vi "MAIN CARICA STRINGHE.vi"() -> ()   [LabVIEW 2019]
uses:
  <vilib>/Utility/file.llb/Read Delimited Spreadsheet (string).vi
panel:
  out "Array":string[](array[string])
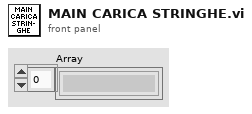
[diagram p1: front panel]
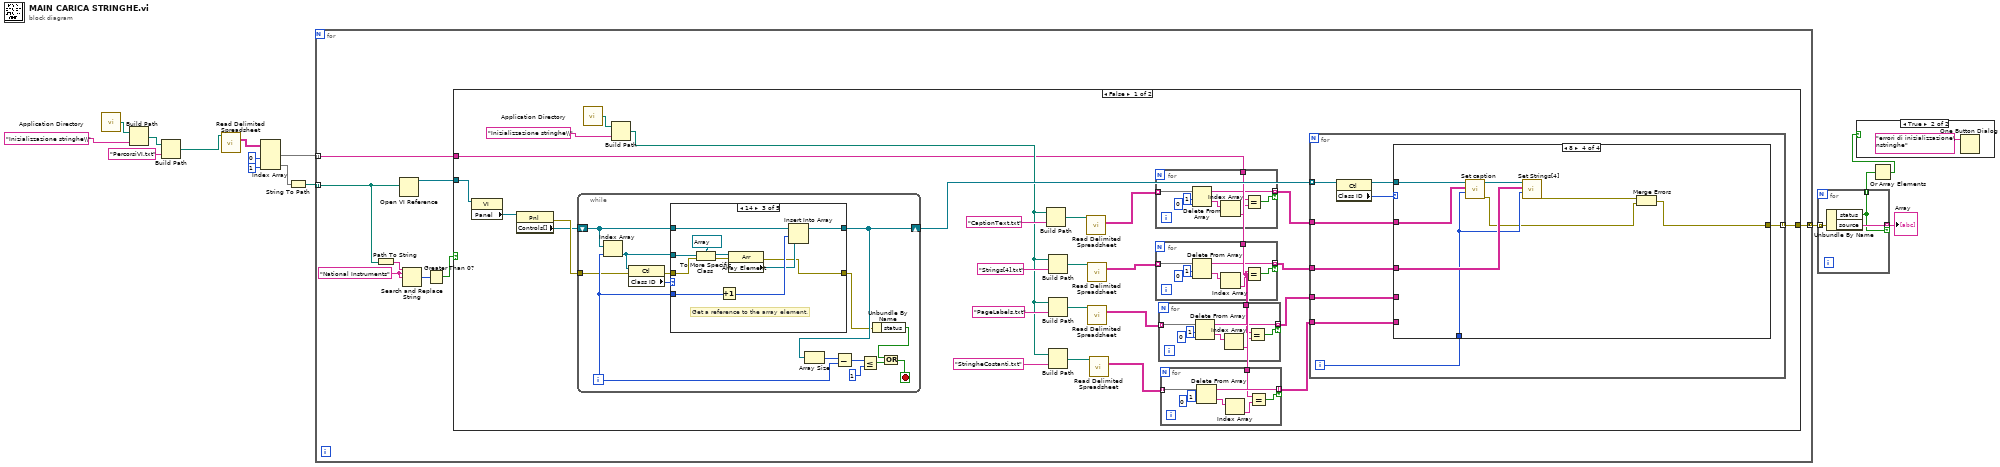
[diagram p0: block diagram]
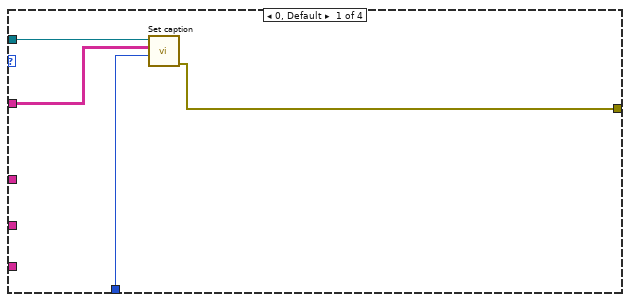
[diagram p3: hidden frame]
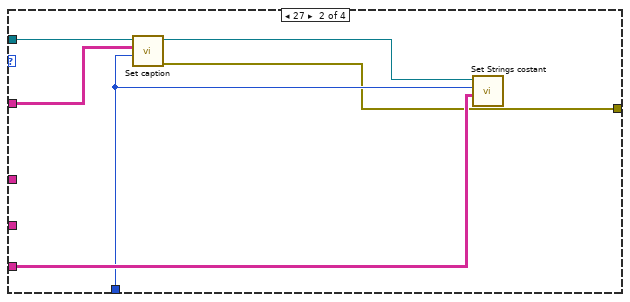
[diagram p4: hidden frame]
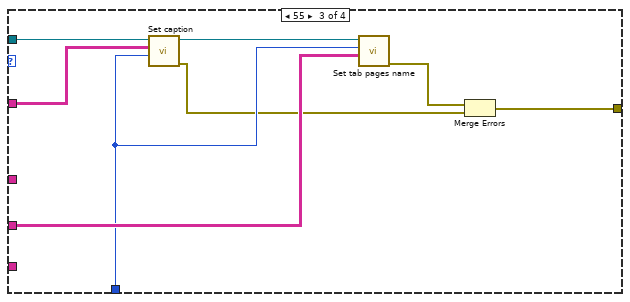
[diagram p5: hidden frame]
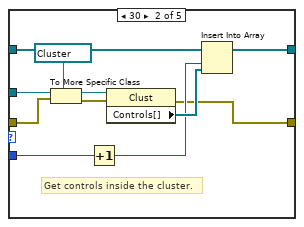
[diagram p7: hidden frame]
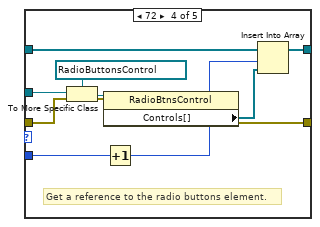
[diagram p8: hidden frame]
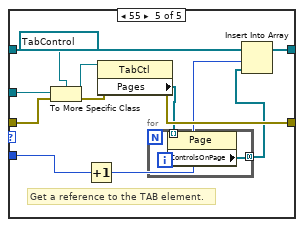
[diagram p9: hidden frame]
diagram:
  n1 = call <vilib>:"Application Directory.vi"() -> ("Application Directory"=w4:path)
  n2 = Build Path(base path=w4, name or relative path="Inizializzazione stringhe\\") -> (appended path=w5:path)
  n3 = Build Path(base path=w5, name or relative path="PercorsiVI.txt") -> (appended path=w6:path)
  n4 = call-poly <vilib>:"Read Delimited Spreadsheet.vi"("file path (dialog if empty)"=w6) -> ("all rows"=w7:string[][])  [unwired: 9 in, 5 out]
  n5 = Index Array(array=w7, index (col) #1=0 ("disabled index (col)"), index (col) #2=1 ("index (col)")) -> (element #1=w10:string[], element #2=w11:string[])  [unwired: 2 in]
  n6 = String To Path(string=w11) -> (path=w12:path[])
  n7 = for {
    tunnel: w12 -> [w21] mode=indexing
    tunnel: w10 -> [w22] mode=indexing
    tunnel: [w16] -> w15 mode=concatenating
    w19 = "National Instruments" ("search string")
    n8 = Path To String(path=w21) -> (string=w20:string)
    n9 = Open VI Reference(vi path=w21) -> (vi reference=w23:refnum<vi>)  [unwired: 5 in, 1 out]
    n10 = Search and Replace String(input string=w20, search string=w19, replace string=w19) -> (number of replacements=w18:i32)  [unwired: 5 in, 3 out]
    n11 = Greater Than 0?(x=w18) -> (x > 0?=w17:bool)
    n12 = case shown="False" w17 {
      tunnel: w23 -> [w46 _]
      tunnel: w22 -> [w24 _]
      tunnel: [w25 _] -> w16
      frame False {
        n13 = property class="VI"(reference=w46) -> ("Panel"=w47:refnum<vi>)  [unwired: 1 in, 2 out]
        n14 = property class="Pnl"(reference=w47) -> (error out=w49:errorcluster, "Controls[]"=w48:refnum<vi>[])  [unwired: 1 in, 1 out]
        n15 = while {
          shift-right: [w121] -> w37
          shift-left: w48 -> [w122]
          tunnel: w49 -> [w120]
          i -> [w127]
          stop <- w125 stop-if-true
          n16 = Index Array(array=w122, index=w127) -> (element=w123:refnum<vi>)
          n17 = property class="Ctl"(reference=w123, error in=w120) -> (error out=w119:errorcluster, "Class ID"=w124:u32)  [unwired: 1 out]
          n18 = case shown="14" w124 {
            tunnel: w123 -> [_ w143 w154 w165 w177]
            tunnel: w122 -> [w132 w140 w151 w164 w176]
            tunnel: w127 -> [_ w139 w150 w163 w175]
            tunnel: [w132 w137 w149 w162 w174] -> w121
            tunnel: w119 -> [w131 w135 w146 w161 w173]
            tunnel: [w131 w133 w144 w160 w172] -> w117
            frame 0, Default {
            }
            frame 30 {
              # "Get controls inside the cluster."
              n19 = To More Specific Class(target class=refnum<vi> refnum ("target class 3"), reference=w143, error in=w135) -> (specific class reference=w142:refnum<vi>, error out=w134:errorcluster)
              n20 = Increment(x=w139) -> (x+1=w136:i32)
              n21 = property class="Clust"(reference=w142, error in=w134) -> (error out=w133:errorcluster, "Controls[]"=w138:refnum<vi>[])  [unwired: 1 out]
              n22 = Insert Into Array(array=w140, index=w136, new element=w138) -> (w137:refnum<vi>[])
            }
            frame 14 {
              # "Get a reference to the array element."
              n23 = To More Specific Class(target class=refnum<vi> refnum ("target class 4"), reference=w154, error in=w146) -> (specific class reference=w153:refnum<vi>, error out=w145:errorcluster)
              n24 = Increment(x=w150) -> (x+1=w148:i32)
              n25 = property class="Arr"(reference=w153, error in=w145) -> (error out=w144:errorcluster, "Array Element"=w147:refnum<vi>)  [unwired: 1 out]
              n26 = Insert Into Array(array=w151, index=w148, new element=w147) -> (w149:refnum<vi>[])
            }
            frame 72 {
              # "Get a reference to the radio buttons element."
              n27 = To More Specific Class(target class=refnum<vi> refnum ("Calcolo P2"), reference=w165, error in=w161) -> (specific class reference=w159:refnum<vi>, error out=w156:errorcluster)
              n28 = property class="RadioBtnsControl"(reference=w159, error in=w156) -> (error out=w160:errorcluster, "Controls[]"=w157:refnum<vi>[])  [unwired: 1 out]
              n29 = Increment(x=w163) -> (x+1=w158:i32)
              n30 = Insert Into Array(array=w164, index=w158, new element=w157) -> (w162:refnum<vi>[])
            }
            frame 55 {
              # "Get a reference to the TAB element."
              n31 = To More Specific Class(target class=refnum<vi> refnum ("Tab Control"), reference=w177, error in=w173) -> (specific class reference=w171:refnum<vi>, error out=w169:errorcluster)
              n32 = Increment(x=w175) -> (x+1=w170:i32)
              n33 = property class="TabCtl"(reference=w171, error in=w169) -> (error out=w172:errorcluster, "Pages"=w167:refnum<vi>[])  [unwired: 1 out]
              n34 = for {
                tunnel: w167 -> [w179] mode=indexing
                tunnel: [w178] -> w166 mode=concatenating
                n35 = property class="Page"(reference=w179) -> ("ControlsOnPage"=w178:refnum<vi>[])  [unwired: 1 in, 2 out]
              }
              n36 = Insert Into Array(array=w176, index=w170, new element=w166) -> (w174:refnum<vi>[])
            }
          }
          n37 = Array Size(array=w121) -> (size(s)=w130:i32)
          n38 = Subtract(x=w130, y=w127) -> (x-y=w129:i32)
          n39 = Less Or Equal?(x=w129, y=1) -> (x <= y?=w126:bool)
          n40 = Unbundle By Name(w117) -> ("status"=w118:bool)
          n41 = Or(x=w118, y=w126) -> (x .or. y?=w125:bool)
        }
        n42 = call <vilib>:"Application Directory.vi"() -> ("Application Directory"=w27:path)
        n43 = Build Path(base path=w27, name or relative path="Inizializzazione stringhe\\") -> (appended path=w26:path)
        n44 = Build Path(base path=w26, name or relative path="CaptionText.txt") -> (appended path=w45:path)
        n45 = Build Path(base path=w26, name or relative path="Strings[4].txt") -> (appended path=w40:path)
        n46 = Build Path(base path=w26, name or relative path="PageLabels.txt") -> (appended path=w39:path)
        n47 = Build Path(base path=w26, name or relative path="StringheCostanti.txt") -> (appended path=w38:path)
        n48 = call-poly <vilib>:"Read Delimited Spreadsheet.vi"("file path (dialog if empty)"=w45) -> ("all rows"=w36:string[][])  [unwired: 9 in, 5 out]
        n49 = call-poly <vilib>:"Read Delimited Spreadsheet.vi"("file path (dialog if empty)"=w40) -> ("all rows"=w34:string[][])  [unwired: 9 in, 5 out]
        n50 = call-poly <vilib>:"Read Delimited Spreadsheet.vi"("file path (dialog if empty)"=w39) -> ("all rows"=w33:string[][])  [unwired: 9 in, 5 out]
        n51 = call-poly <vilib>:"Read Delimited Spreadsheet.vi"("file path (dialog if empty)"=w38) -> ("all rows"=w32:string[][])  [unwired: 9 in, 5 out]
        n52 = for {
          tunnel: w36 -> [w81] mode=indexing
          tunnel: [w77] -> w35 mode=indexing if=w75
          tunnel: w24 -> [w74]
          n53 = Delete From Array(array=w81, length=1, index=0) -> (deleted portion=w78:string[], array with subset deleted=w77:string[])
          n54 = Index Array(array=w78) -> (element=w76:string)  [unwired: 1 in]
          n55 = Equal?(x=w74, y=w76) -> (x = y?=w75:bool)
        }
        n56 = for {
          tunnel: w34 -> [w73] mode=indexing
          tunnel: [w69] -> w31 mode=indexing if=w67
          tunnel: w24 -> [w66]
          n57 = Delete From Array(array=w73, length=1, index=0) -> (deleted portion=w70:string[], array with subset deleted=w69:string[])
          n58 = Index Array(array=w70) -> (element=w68:string)  [unwired: 1 in]
          n59 = Equal?(x=w66, y=w68) -> (x = y?=w67:bool)
        }
        n60 = for {
          tunnel: w33 -> [w65] mode=indexing
          tunnel: [w61] -> w30 mode=indexing if=w59
          tunnel: w24 -> [w58]
          n61 = Delete From Array(array=w65, length=1, index=0) -> (deleted portion=w62:string[], array with subset deleted=w61:string[])
          n62 = Index Array(array=w62) -> (element=w60:string)  [unwired: 1 in]
          n63 = Equal?(x=w58, y=w60) -> (x = y?=w59:bool)
        }
        n64 = for {
          tunnel: w32 -> [w57] mode=indexing
          tunnel: [w53] -> w29 mode=indexing if=w51
          tunnel: w24 -> [w50]
          n65 = Delete From Array(array=w57, length=1, index=0) -> (deleted portion=w54:string[], array with subset deleted=w53:string[])
          n66 = Index Array(array=w54) -> (element=w52:string)  [unwired: 1 in]
          n67 = Equal?(x=w50, y=w52) -> (x = y?=w51:bool)
        }
        n68 = for {
          tunnel: w35 -> [w87]
          tunnel: w31 -> [w86]
          tunnel: w37 -> [w90] mode=indexing
          tunnel: w30 -> [w84]
          tunnel: w29 -> [w83]
          tunnel: [w82] -> w25 mode=indexing
          i -> [w85]
          n69 = property class="Ctl"(reference=w90) -> (reference out=w88:refnum<vi>, "Class ID"=w89:u32)  [unwired: 1 in, 1 out]
          n70 = case shown="8" w89 {
            tunnel: w88 -> [w94 w100 w108 w115]
            tunnel: w87 -> [w93 w99 w107 w113]
            tunnel: w86 -> [_ _ _ w116]
            tunnel: w85 -> [w92 w96 w104 w112]
            tunnel: w84 -> [_ _ w105 _]
            tunnel: w83 -> [_ w97 _ _]
            tunnel: [w91 w95 w101 w109] -> w82
            frame 0, Default {
              n71 = call "Set caption.vi"("index (row)"=w92, "Array"=w93, "Control in"=w94) -> ("error out"=w91:errorcluster)  [unwired: 7 in, 1 out]
            }
            frame 27 {
              n72 = call "Set caption.vi"("index (row)"=w96, "Array"=w99, "Control in"=w100) -> ("error out"=w95:errorcluster, "reference out"=w98:refnum<vi>)  [unwired: 7 in]
              n73 = call "Set Strings costant.vi"("all rows"=w97, "Numeric"=w96, "Control in"=w98) -> ()  [unwired: 9 in]
            }
            frame 55 {
              n74 = call "Set caption.vi"("index (row)"=w104, "Array"=w107, "Control in"=w108) -> ("error out"=w102:errorcluster, "reference out"=w106:refnum<vi>)  [unwired: 7 in]
              n75 = call "Set tab pages name.vi"("Array"=w105, "Numeric"=w104, "Control in"=w106) -> ("error out"=w103:errorcluster)  [unwired: 7 in, 1 out]
              n76 = Merge Errors(w103, w102) -> (w101:errorcluster)
            }
            frame 8 {
              n77 = call "Set caption.vi"("index (row)"=w112, "Array"=w113, "Control in"=w115) -> ("error out"=w110:errorcluster, "reference out"=w114:refnum<vi>)  [unwired: 7 in]
              n78 = call "Set Strings[4].vi"("index (row)"=w112, "Array"=w116, "Control in"=w114) -> ("error out"=w111:errorcluster)  [unwired: 7 in, 1 out]
              n79 = Merge Errors(w111, w110) -> (w109:errorcluster)
            }
          }
        }
      }
      frame True {
        # "scarta i vi nella cartella national instruments (quelli della libreria labview)"
      }
    }
  }
  n80 = for {
    tunnel: w15 -> [w182] mode=indexing
    tunnel: [w181] -> w1 mode=indexing if=w180
    tunnel: [w180] -> w14 mode=indexing
    n81 = Unbundle By Name(w182) -> ("status"=w180:bool, "source"=w181:string)
  }
  "Array" <- w1
  n82 = Or Array Elements(Boolean array=w14) -> (logical OR=w13:bool)
  n83 = case shown="True" w13 {
    frame False {
    }
    frame True {
      n84 = One Button Dialog(message="errori di inizializzazione\nstringhe") -> ()  [unwired: 1 in, 1 out]
    }
  }
